vi "ConsolidatedLimitSwitch.vi"(8 "CurrentLSValue":bool, 9 "LastLSValue":bool, 10 "CurrentInput":dbl, 11 "LastSign":dbl) -> (1 "NewSign":dbl, 2 "RelayValue":T1)   [LabVIEW 2012]
doc: "For use with coupled limit switches. Detects sign of input, maintains that, and blocks all input in that direction. Outputs relay signal. Requires LastSign and LastLSValue to be maintained by shift register in outside loop. Results unexpected when given 0 for CurrentInput."
uses:
  <vilib>/Rock Robotics/WPI/Relay/WPI_RelayValue.ctl
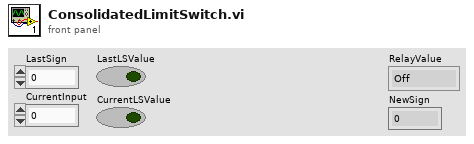
[diagram p1: front panel]
types:
  T1 = typedef "WPI_RelayValue.ctl" = enum16{"Off", "On", "Forward", "Reverse"}
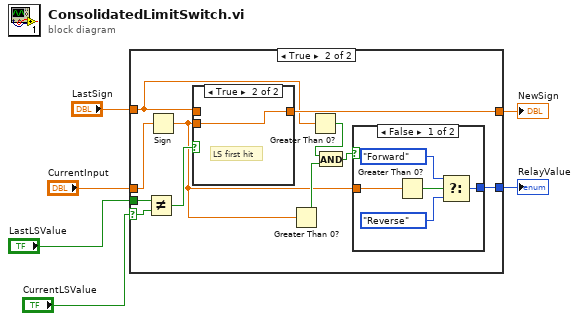
[diagram p0: block diagram]
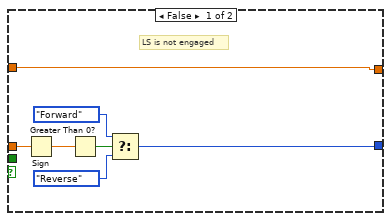
[diagram p2: hidden frame]
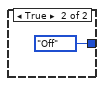
[diagram p3: hidden frame]
diagram:
  n1 = case shown="True" "CurrentLSValue" {
    selector: "CurrentLSValue" -> [_ w24]
    tunnel: "CurrentInput" -> [w13 w19]
    tunnel: [w8 w21] -> w2
    tunnel: "LastLSValue" -> [_ w23]
    tunnel: "LastSign" -> [w7 w18]
    tunnel: [w7 w20] -> w1
    frame False {
      # "LS is not engaged"
      n2 = Sign(1:w13) -> (0:w12:dbl)
      n3 = Greater Than 0?(x=w12) -> (x > 0?=w11:bool)
      n4 = Select(t=WPI_RelayValue."Forward" ("RelayValue"), s=w11, f=WPI_RelayValue."Reverse") -> (s? t:f=w8:T1)
    }
    frame True {
      n5 = Not Equal?(x=w23, y=w24) -> (x != y?=w22:bool)
      n6 = Sign(1:w19) -> (0:w14:dbl)
      n7 = case shown="True" w22 {
        tunnel: w18 -> [w31 _]
        tunnel: w14 -> [_ w32]
        tunnel: [w31 w32] -> w20
        frame False {
          # "LS is still\nengaged"
        }
        frame True {
          # "LS first hit"
        }
      }
      n8 = Greater Than 0?(x=w14) -> (x > 0?=w17:bool)
      n9 = Greater Than 0?(x=w18) -> (x > 0?=w16:bool)
      n10 = And(x=w16, y=w17) -> (x .and. y?=w15:bool)
      n11 = case shown="False" w15 {
        tunnel: [w25 WPI_RelayValue."Off" ("RelayValue")] -> w21
        tunnel: w14 -> [w26 _]
        frame False {
          n12 = Greater Than 0?(x=w26) -> (x > 0?=w27:bool)
          n13 = Select(t=WPI_RelayValue."Forward" ("RelayValue"), s=w27, f=WPI_RelayValue."Reverse") -> (s? t:f=w25:T1)
        }
        frame True {
        }
      }
    }
  }
  "RelayValue" <- w2
  "NewSign" <- w1
